vi "AddSubscriber.vi"(0 "object in":refnum<class "EmergencyController.lvclass">, 2 "EmergancyStopObject":refnum<class>, 5 "error in (no error)":errorcluster) -> (14 "object out":refnum<class "EmergencyController.lvclass">, 19 "error out":errorcluster)   [LabVIEW 2014, in "EmergencyController.lvclass"]
uses:
  EmergencyController.lvclass
  EmergencyController.lvclass/EmergencyController.ctl
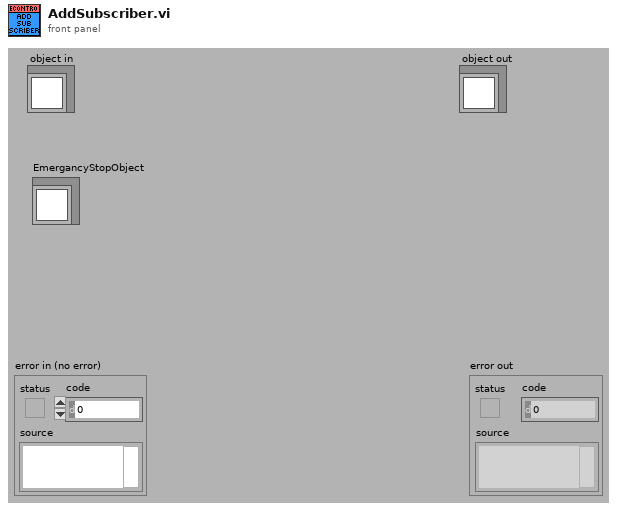
[diagram p1: front panel]
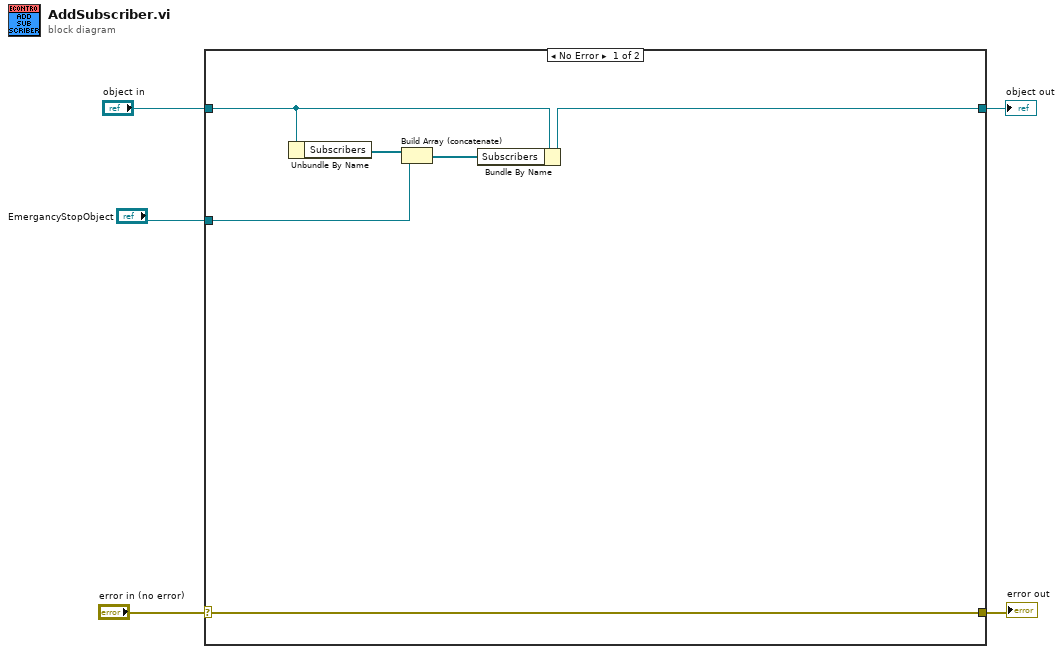
[diagram p0: block diagram]
diagram:
  n1 = case shown="No Error" "error in (no error)" {
    selector: "error in (no error)" -> [w11 w13]
    tunnel: [w11 w13] -> w4
    tunnel: [w7 w12] -> w2
    tunnel: "object in" -> [w10 w12]
    tunnel: "EmergancyStopObject" -> [w8 _]
    frame No Error {
      n2 = Unbundle By Name(w10) -> ("Subscribers"=w9:refnum<class>[])
      n3 = Build Array (concatenate)(w9, w8) -> (w6:refnum<class>[])
      n4 = Bundle By Name(cluster=w10, "Subscribers"=w6) -> (w7:refnum<class "EmergencyController.lvclass">)
    }
    frame Error {
    }
  }
  "error out" <- w4
  "object out" <- w2
